vi "Adapt To Type.vi"(7 "Type and Defaults":variant, 8 "error in (no error)":errorcluster, 10 "Variant in":variant, 11 "Deserializer in":refnum<class "Deserializer.lvclass">) -> (0 "error out":errorcluster, 2 "Variant out":variant, 3 "Deserializer out":refnum<class "Deserializer.lvclass">)   [LabVIEW 2020, in "JKI JSON Object Serialization.lvlib" / "Deserializer.lvclass"]
doc: "Adapts <b>Variant in</b> previously unflattened from a JSON formatted string to match the type of <b>Type and Defaults</b>. For any cluster element in Type and Defaults, the value of the element in Type and Default is used if element with the same name is not present in Variant in. \n\nGCraftsman JSON Object Serialization Toolkit\nwww.GCraftsman.com\nCopyright (c) 2017, GCraftsman"
uses:
  Deserializer.lvclass
  Support/OOP_Utility/Reflection/getObjectPrivateData.vi
  Support/OOP_Utility/Reflection/Assert No Duplicate Named Private Data Elements.vi
  Support/OOP_Utility/Reflection/Assert No Duplicate Named Private Data Elements.vi/91249ab7-5ea3-4d6c-b8df-29db4c9f394f.vi
  Support/OOP_Utility/Reflection/Assert No Duplicate Named Private Data Elements.vi/f7c1a62c-1232-4a35-ba9e-0fa75d385864.vi
  <vilib>/AdvancedString/1D String Array to Delimited String.vi
  <vilib>/dlg_ctls.llb/Space Constant.vi
  Support/OOP_Utility/Reflection/Assert No Duplicate Named Private Data Elements.vi/91249ab7-5ea3-4d6c-b8df-29db4c9f394f.vi/73eff78f-802f-4e82-99e6-5ec6d44c8b1c.vi
  Support/OOP_Utility/Reflection/Assert No Duplicate Named Private Data Elements.vi/91249ab7-5ea3-4d6c-b8df-29db4c9f394f.vi/a79ef678-9021-4176-8e9d-ef71acec083e.vi
  Support/OOP_Utility/Reflection/Assert No Duplicate Named Private Data Elements.vi/91249ab7-5ea3-4d6c-b8df-29db4c9f394f.vi/6194b64b-8f19-4369-9ca4-18e99c56e175.vi
  Support/OOP_Utility/Reflection/Assert No Duplicate Named Private Data Elements.vi/91249ab7-5ea3-4d6c-b8df-29db4c9f394f.vi/4000f349-3ba7-45cd-93a4-b1a8967d5605.vi
  <vilib>/Utility/LVClass/Get LV Class Name.vi
  Support/OOP_Utility/Reflection/reflectionPool.vi
  <userlib>/_OpenG.lib/lvdata/lvdata.llb/Get Cluster Element Names__ogtk.vi
  <vilib>/Utility/error.llb/Error Cluster From Error Code.vi
  <userlib>/_OpenG.lib/lvdata/lvdata.llb/Array of VData to VCluster__ogtk.vi
  <vilib>/addons/_JKI.lib/Serialization/JSON/Deserializer/JSON Deserializer/JSON Deserializer.lvclass
  Deserializer.lvclass/Deserializer.ctl
  Support/OOP_Utility/OOP_Utility.lvlib
  <vilib>/Utility/Data Type/NI_Data Type.lvlib
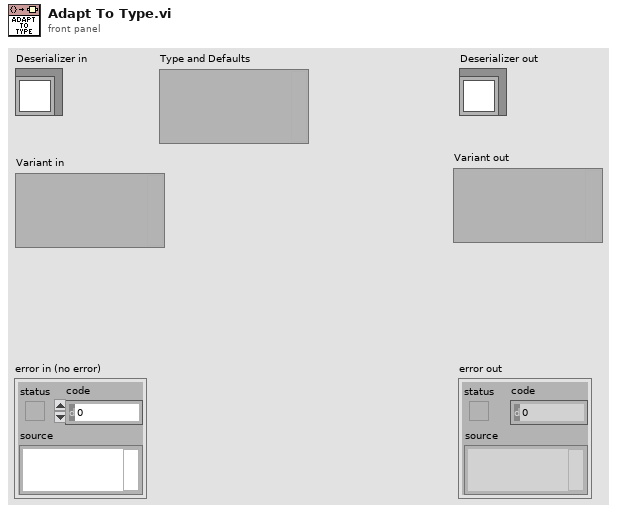
[diagram p1: front panel]
types:
  T1 = typedef "NI_Data Type.lvlib/Data Type.ctl" = enum8{"Invalid Type", "Void", "I8", "I16", "I32", "I64", "U8", "U16", "U32", "U64", "Single Float", "Double Float", "Extended Float", "Single Complex", "Double Complex", "Extended Complex", "Enum U8", "Enum U16", "Enum U32", "Enum U64", "Single Float With Unit", "Double Float With Unit", "Extended Float With Unit", "Single Complex with Unit", "Double Complex with Unit", "Extended Complex with Unit", "Boolean", "String", "Path", "Picture", "Tag", "Array", "Cluster", "Variant", "LV Variant", "Waveform", "Timestamp", "Digital Waveform", "Digital Data", "ExpressData", "Refnum", "External Data", "VI", "Poly VI", "LabVIEW Class Instance", "Fixed Point", "Set Collection", "Map Collection"}
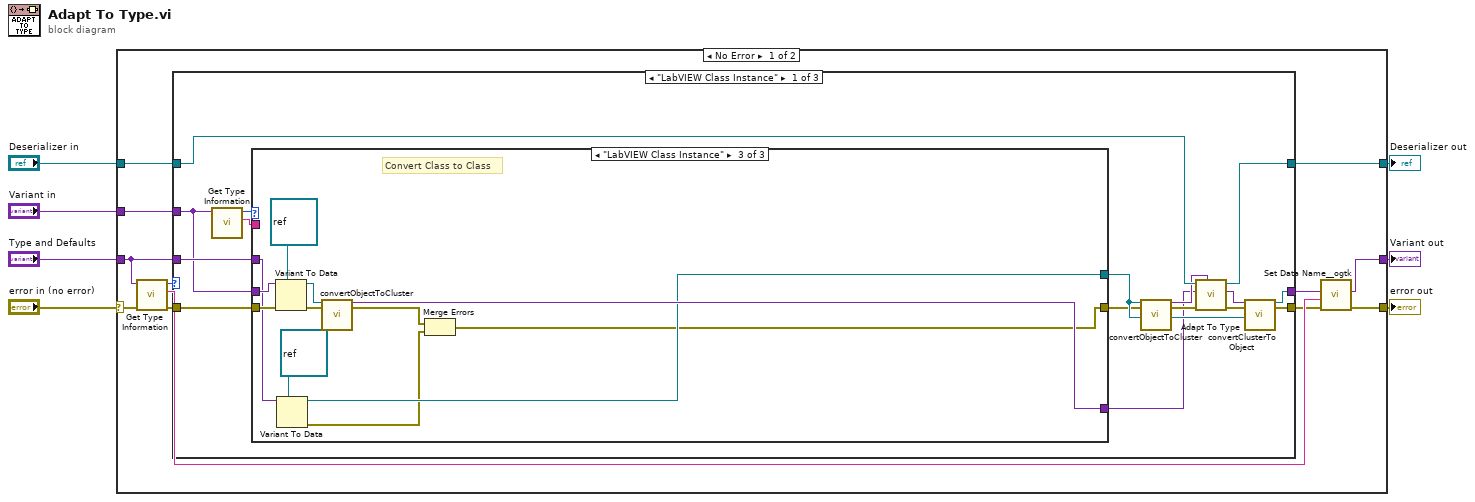
[diagram p0: block diagram]
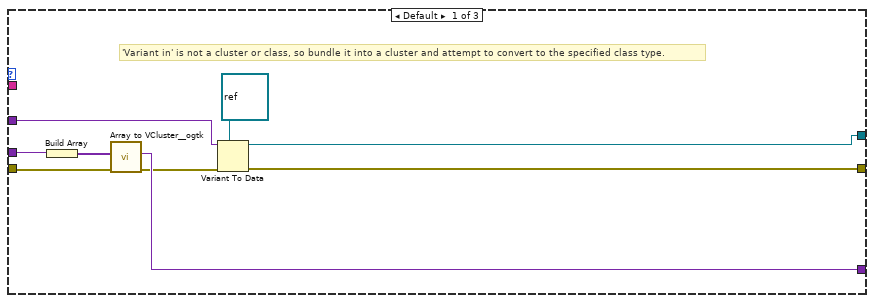
[diagram p2: hidden frame]
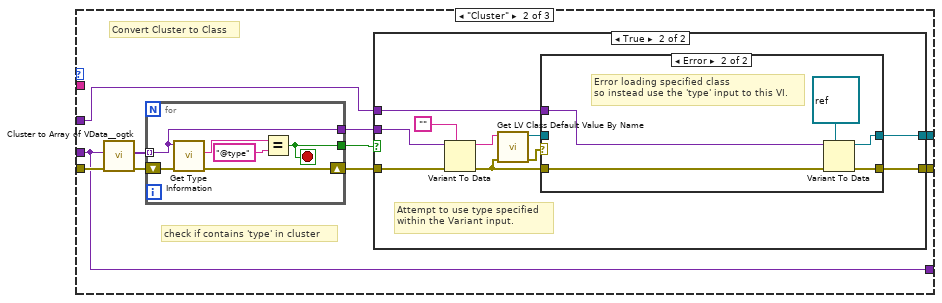
[diagram p3: hidden frame]
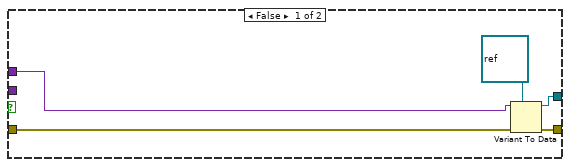
[diagram p4: hidden frame]
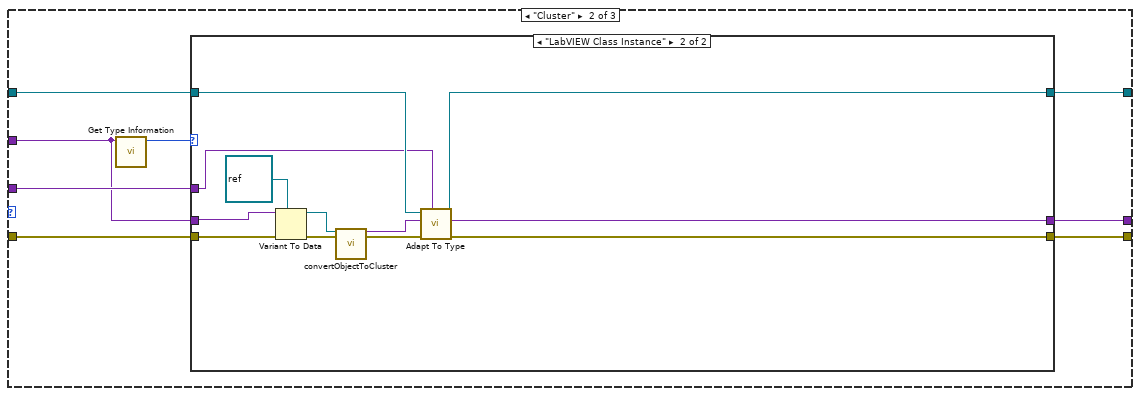
[diagram p6: hidden frame]
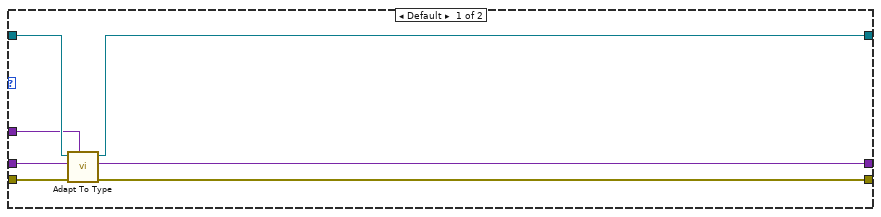
[diagram p7: hidden frame]
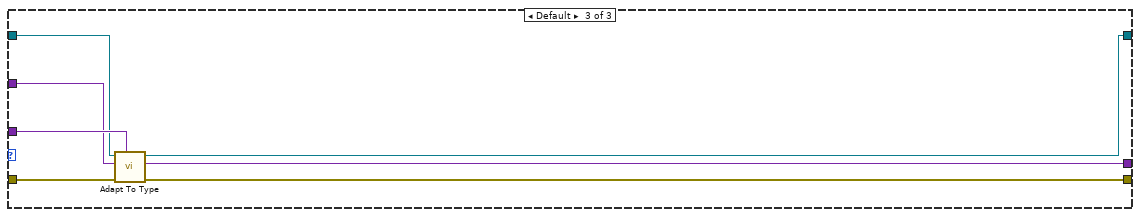
[diagram p8: hidden frame]
diagram:
  n1 = case shown="No Error" "error in (no error)" {
    selector: "error in (no error)" -> [w19 w129]
    tunnel: [w9 w129] -> w7
    tunnel: [w12 w130] -> w6
    tunnel: [w14 w131] -> w5
    tunnel: "Type and Defaults" -> [w15 w130]
    tunnel: "Variant in" -> [w8 _]
    tunnel: "Deserializer in" -> [w18 w131]
    frame No Error {
      n2 = call <vilib>:"Get Type Information.vi"("error in (no error)"=w19, "variant"=w15) -> ("error out"=w17:errorcluster, "name"=w11:string, "type"=w16:T1)  [unwired: 5 in, 2 out]
      n3 = case shown="\"LabVIEW Class Instance\"" w16 {
        tunnel: [w35 w96 w128] -> w10
        tunnel: [w34 w95 w127] -> w13
        tunnel: [w32 w100 w126] -> w14
        tunnel: w15 -> [w24 w99 w125]
        tunnel: w18 -> [w33 w101 w124]
        tunnel: w17 -> [w26 w97 w123]
        tunnel: w8 -> [w22 w98 w122]
        frame "LabVIEW Class Instance" {
          n4 = call <vilib>:"Get Type Information.vi"("variant"=w22) -> ("name"=w20:string, "type"=w23:T1)  [unwired: 6 in, 3 out]
          n5 = case shown="\"Cluster\"" w23 {
            tunnel: [w36 w54 w85] -> w29
            tunnel: w26 -> [w41 w51 w90]
            tunnel: [w37 w48 w83] -> w25
            tunnel: w24 -> [w39 w47 w89]
            tunnel: w22 -> [w43 w45 w91]
            tunnel: [w42 w45 w87] -> w21
            tunnel: w20 -> [_ _ _]
            frame Default {
              # "'Variant in' is not a cluster or class, so bundle it into a cluster and attempt to convert to the specified class type."
              n6 = Build Array(w43) -> (w44:variant[])
              n7 = call <userlib>:"Array to VCluster__ogtk.vi"("error in (no error)"=w41, "Array"=w44) -> ("error out"=w38:errorcluster, "VCluster"=w42:variant)  [unwired: 8 in]
              n8 = Variant To Data(error in=w38, type=refnum<class> refnum ("LabVIEW Object"), Variant=w39) -> (data=w36:refnum<class>, error out=w37:errorcluster)
            }
            frame "Cluster" {
              # "check if contains 'type' in cluster"
              # "Convert Cluster to Class"
              n9 = call <userlib>:"Cluster to Array of VData__ogtk.vi"("error in (no error)"=w51, "Cluster"=w45) -> ("error out"=w50:errorcluster, "Array of VData"=w52:variant[])  [unwired: 8 in]
              n10 = for {
                tunnel: w52 -> [w55] mode=indexing
                shift-right: [w59] -> w46
                shift-left: w50 -> [w60]
                tunnel: [w56] -> w53
                tunnel: [w55] -> w49
                stop <- w56 stop-if-true
                n11 = call <vilib>:"Get Type Information.vi"("error in (no error)"=w60, "variant"=w55) -> ("error out"=w59:errorcluster, "name"=w58:string)  [unwired: 5 in, 3 out]
                n12 = Equal?(x=w58, y="@type") -> (x = y?=w56:bool)
              }
              n13 = case shown="True" w53 {
                tunnel: [w61 w74] -> w54
                tunnel: w49 -> [_ w71]
                tunnel: w46 -> [w63 w72]
                tunnel: [w62 w68] -> w48
                tunnel: w47 -> [w65 w66]
                frame False {
                  n14 = Variant To Data(error in=w63, type=refnum<class> refnum ("LabVIEW Object"), Variant=w65) -> (data=w61:refnum<class>, error out=w62:errorcluster)
                }
                frame True {
                  # "Attempt to use type specified\nwithin the Variant input."
                  n15 = Variant To Data(error in=w72, type="", Variant=w71) -> (data=w70:string, error out=w67:errorcluster)
                  n16 = call <vilib>:"Get LV Class Default Value By Name.vi"("error in (no error)"=w67, "class name"=w70) -> ("error out"=w69:errorcluster, "object"=w75:refnum<class>)  [unwired: 8 in]
                  n17 = case shown="No Error" w69 {
                    tunnel: w75 -> [w77 _]
                    tunnel: [w77 w80] -> w74
                    tunnel: [w76 w78] -> w68
                    tunnel: w67 -> [w76 w79]
                    tunnel: w66 -> [_ w81]
                    frame No Error {
                    }
                    frame Error {
                      # "Error loading specified class\nso instead use the 'type' input to this VI."
                      n18 = Variant To Data(error in=w79, type=refnum<class> refnum ("LabVIEW Object"), Variant=w81) -> (data=w80:refnum<class>, error out=w78:errorcluster)
                    }
                  }
                }
              }
            }
            frame "LabVIEW Class Instance" {
              # "Convert Class to Class"
              n19 = Variant To Data(error in=w90, type=refnum<class> refnum ("LabVIEW Object"), Variant=w91) -> (data=w93:refnum<class>, error out=w94:errorcluster)
              n20 = Variant To Data(type=refnum<class> refnum ("LabVIEW Object"), Variant=w89) -> (data=w85:refnum<class>, error out=w84:errorcluster)  [unwired: 1 in]
              n21 = call "convertObjectToCluster.vi"("Object in"=w93, "error in"=w94) -> ("VCluster"=w87:variant, "error out"=w86:errorcluster)  [unwired: 16 in]
              n22 = Merge Errors(w86, w84) -> (w83:errorcluster)
            }
          }
          n23 = call "convertObjectToCluster.vi"("Object in"=w29, "error in"=w25) -> ("VCluster"=w28:variant, "error out"=w30:errorcluster)  [unwired: 16 in]
          n24 = call-parent "Adapt To Type.vi"("Type and Defaults"=w28, "error in (no error)"=w30, "Variant in"=w21, "Deserializer in"=w33) -> ("error out"=w31:errorcluster, "Variant out"=w27:variant, "Deserializer out"=w32:refnum<class "Deserializer.lvclass">)  [unwired: 5 in]
          n25 = call "convertClusterToObject.vi"("clusterData"=w27, "error in"=w31, "objectType"=w29) -> ("object out"=w34:refnum<class>, "error out"=w35:errorcluster)  [unwired: 15 in]
        }
        frame "Cluster" {
          n26 = call <vilib>:"Get Type Information.vi"("variant"=w98) -> ("type"=w102:T1)  [unwired: 6 in, 4 out]
          n27 = case shown="\"LabVIEW Class Instance\"" w102 {
            tunnel: w101 -> [w109 w115]
            tunnel: [w108 w111] -> w100
            tunnel: w99 -> [w107 w114]
            tunnel: w98 -> [w106 w119]
            tunnel: w97 -> [w105 w120]
            tunnel: [w104 w112] -> w96
            tunnel: [w103 w110] -> w95
            frame Default {
              n28 = call-parent "Adapt To Type.vi"("Type and Defaults"=w107, "error in (no error)"=w105, "Variant in"=w106, "Deserializer in"=w109) -> ("error out"=w104:errorcluster, "Variant out"=w103:variant, "Deserializer out"=w108:refnum<class "Deserializer.lvclass">)  [unwired: 5 in]
            }
            frame "LabVIEW Class Instance" {
              n29 = Variant To Data(error in=w120, type=refnum<class> refnum ("objectType"), Variant=w119) -> (data=w118:refnum<class>, error out=w117:errorcluster)
              n30 = call "convertObjectToCluster.vi"("Object in"=w118, "error in"=w117) -> ("VCluster"=w116:variant, "error out"=w113:errorcluster)  [unwired: 16 in]
              n31 = call-parent "Adapt To Type.vi"("Type and Defaults"=w114, "error in (no error)"=w113, "Variant in"=w116, "Deserializer in"=w115) -> ("error out"=w112:errorcluster, "Variant out"=w110:variant, "Deserializer out"=w111:refnum<class "Deserializer.lvclass">)  [unwired: 5 in]
            }
          }
        }
        frame Default {
          n32 = call-parent "Adapt To Type.vi"("Type and Defaults"=w125, "error in (no error)"=w123, "Variant in"=w122, "Deserializer in"=w124) -> ("error out"=w128:errorcluster, "Variant out"=w127:variant, "Deserializer out"=w126:refnum<class "Deserializer.lvclass">)  [unwired: 5 in]
        }
      }
      n33 = call <userlib>:"Set Data Name__ogtk.vi"("error in (no error)"=w10, "Data Name"=w11, "Data"=w13) -> ("error out"=w9:errorcluster, "Renamed Data"=w12:variant)  [unwired: 7 in]
    }
    frame Error {
    }
  }
  "error out" <- w7
  "Deserializer out" <- w5
  "Variant out" <- w6
